vi "Read Type.vi"(8 "error in (no error)":errorcluster, 11 "Termination in":refnum<class "Termination.lvclass">) -> (0 "error out":errorcluster, 2 "Enum":T1, 3 "Termination out":refnum<class "Termination.lvclass">)   [LabVIEW 2020, in "Termination.lvclass"]
uses:
  Termination.lvclass
  Typedefs/Tosca-Event Type.ctl
  Termination.lvclass/Termination.ctl
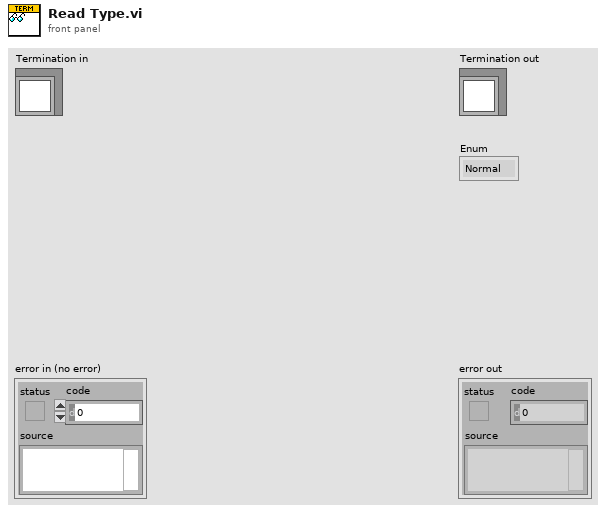
[diagram p1: front panel]
types:
  T1 = typedef "Tosca-Event Type.ctl" = enum16{"Normal", "CS+", "CS-"}
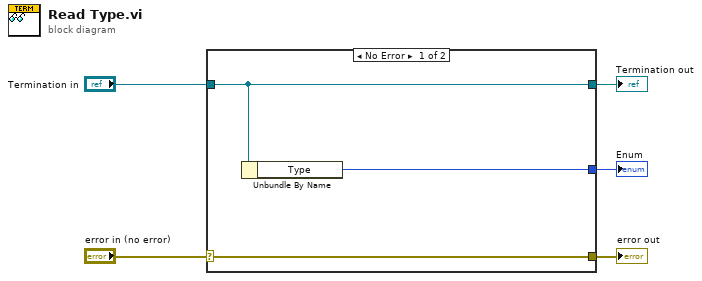
[diagram p0: block diagram]
diagram:
  n1 = case shown="No Error" "error in (no error)" {
    selector: "error in (no error)" -> [w8 w9]
    tunnel: [w8 w9] -> w4
    tunnel: [w7 w10] -> w2
    tunnel: "Termination in" -> [w7 w10]
    tunnel: [w6 _] -> w1
    frame No Error {
      n2 = Unbundle By Name(w7) -> ("Type"=w6:T1)
    }
    frame Error {
    }
  }
  "error out" <- w4
  "Termination out" <- w2
  "Enum" <- w1
